vi "rs3 Get_calibration_table.vi"(8 "error in (no error)":errorcluster, 11 "Device in":u64) -> (0 "error out":errorcluster, 1 "error":u64, 2 "PointerToOldCalibrationTable":u64, 3 "Device out":u64)   [LabVIEW 2017, in "libRealSense3.lvlib"]
doc: "STARTS the streaming of a specific sensor, based on the input QUEUE."
uses:
  libRealSense3.lvlib
  realsense2.dll
panel:
  # "RS Get Calibration Table"
  # "(C) 2019 Intel Corp.,  AGJ"
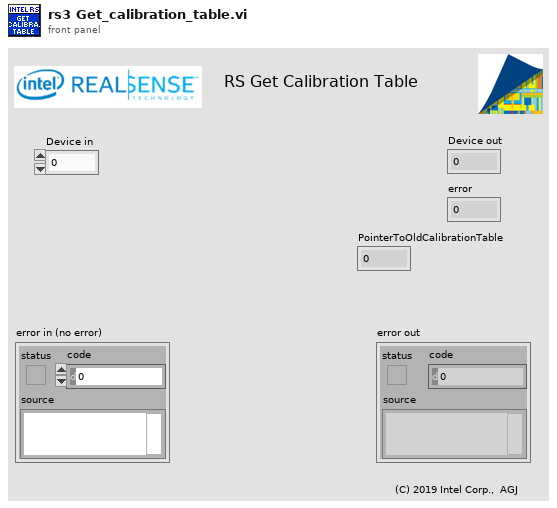
[diagram p1: front panel]
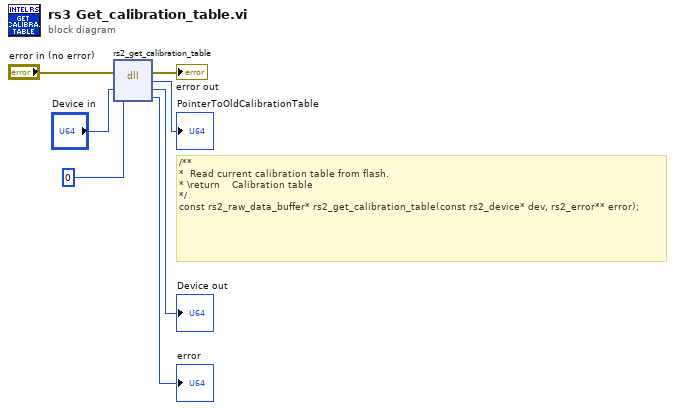
[diagram p0: block diagram]
diagram:
  # "/**\n*  Read current calibration table from flash.\n* \\return    Calibration table\n*/\nconst rs2_raw_data_buffer* rs2_get_calibration_table(const rs2_device* dev, rs2_error** error);"
  n1 = dll-call lib="C:/Users/agrunnet/Documents/libRealSense6/realsense2.dll" fn="rs2_get_calibration_table"(error in="error in (no error)", "device"="Device in", "error"=u64 0) -> (error out=→"error out":errorcluster, "OldcalibrationTable"=→"PointerToOldCalibrationTable":u64, "device"=→"Device out":u64, "error"=→"error":u64)  [unwired: 2 in, 1 out]
